vi "DrawImageToPictureARGB.vi"(7 "Image Draw Offset (Default 0,0)":T1, 8 "error in (no error)":errorcluster, 11 "ARGB Image Source":refnum<data-value>) -> (0 "error out":errorcluster, 3 "Picture":picture)   [LabVIEW 2020, in "g_ar_toolkit.image.lvlib"]
uses:
  g_ar_toolkit.image.lvlib
  8cd07b1b-062e-4fe4-9e87-2eb3dc89fe0e.vi
  Image Draw Offset.ctl
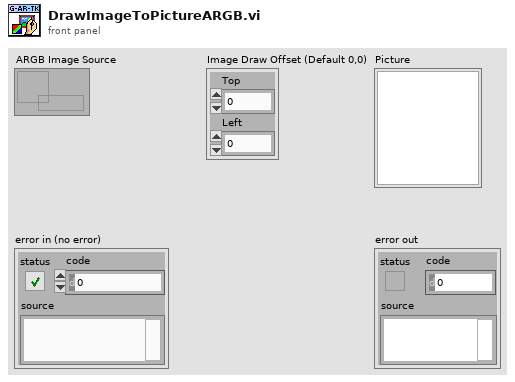
[diagram p1: front panel]
types:
  T1 = typedef "g_ar_toolkit.image.lvlib/Image Draw Offset.ctl" = cluster{"Top":i16, "Left":i16}
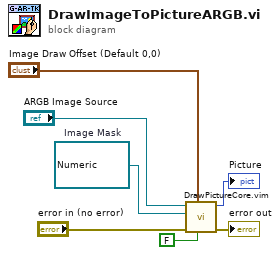
[diagram p0: block diagram]
diagram:
  w1 = refnum<data-value> refnum  # Image Mask
  n1 = call "DrawPictureCore.vim"("HasMask"=FALSE, "Image Draw Offset"="Image Draw Offset (Default 0,0)", "error in (no error)"="error in (no error)", "Image Mask"=w1, "Image Src"="ARGB Image Source") -> ("error out"=→"error out":errorcluster, "Picture"=→"Picture":picture)  [unwired: 5 in]
